vi "Sync2Tekron.vi"(0 "instrument handle in":refnum<k15>, 1 "error in (no error)":errorcluster) -> (7 "instrument handle out":refnum<k15>, 8 "error out":errorcluster, 9 "Synchronized":bool, 10 "Grandmaster Clock ID":string)   [LabVIEW 2021]
panel:
  in  "BMCA Mode":i32(ring) items=["SlaveOnly", "MasterSlave"]
  in  "1588:Clock Accuracy":i32(ring) items=["Unknown", "Within25nsec", "Within100nsec", "Within250nsec", "Within1usec", "Within2500nsec", "Within10usec", "Within25usec", "Within100usec", "Within250usec", "Within1msec", "Within2500usec", "Within10msec", "Within25msec", "Within100msec", "Within250msec", "Within1sec", "Within10sec", "GreaterThan10sec"]
  in  "Clock State":i32(ring) items=["Initializing", "Faulty", "Disabled", "Listening", "PreMaster", "Master", "Passive", "Uncalibrated", "Slave", "Stopped"]
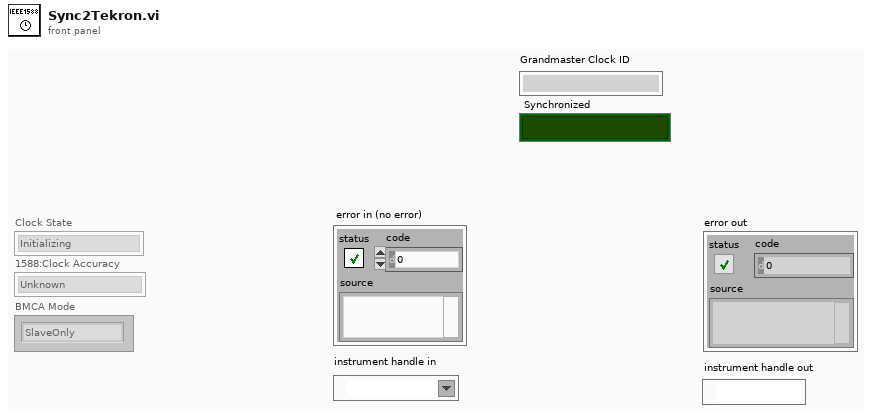
[diagram p1: front panel]
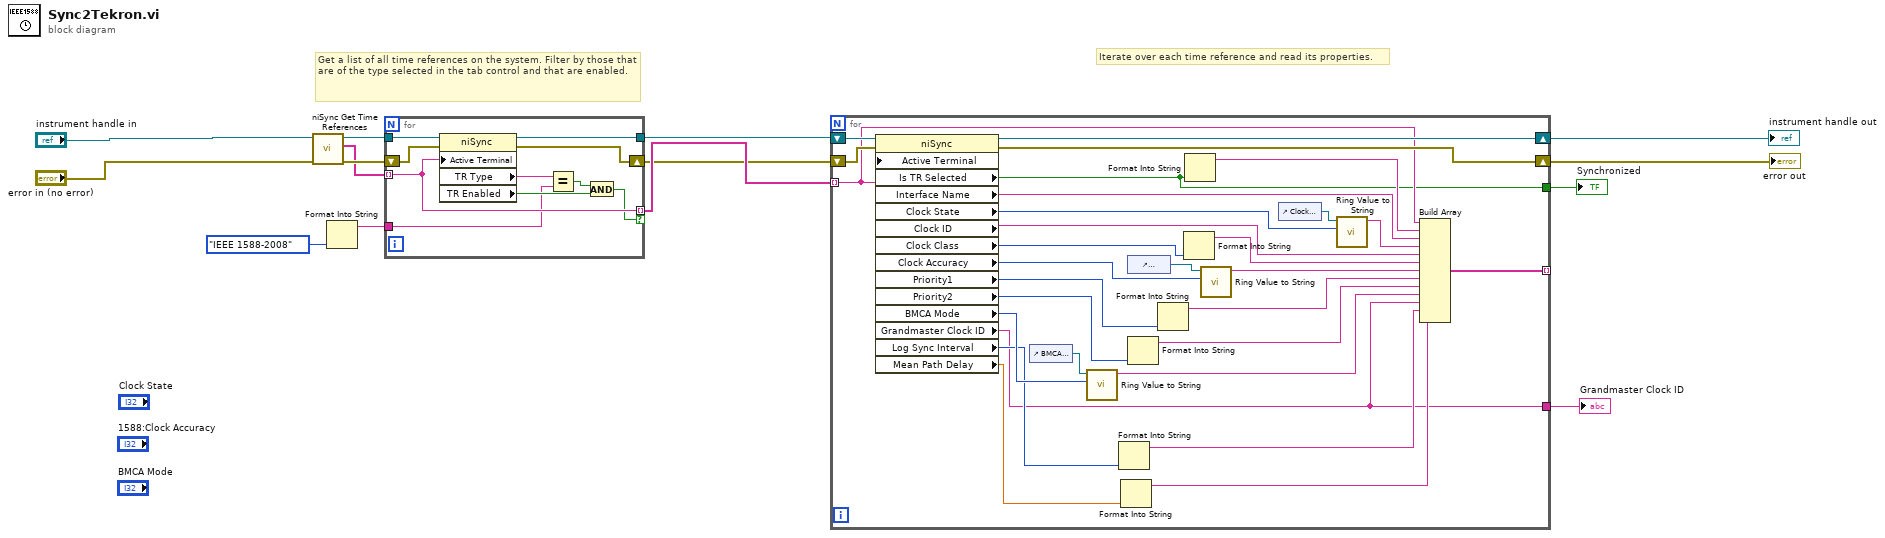
[diagram p0: block diagram]
diagram:
  # "Iterate over each time reference and read its properties."
  # "Get a list of all time references on the system. Filter by those that are of the type selected in the tab control and that are enabled."
  n1 = call <instrlib>:"niSync Get Time References.vi"("error in (no error)"="error in (no error)", "instrument handle"="instrument handle in") -> ("error out"=w13:errorcluster, "time references"=w12:string[], "instrument handle out"=w14:refnum<k15>)  [unwired: 7 in]
  n2 = Format Into String(enum32{"IEEE 1588-2008", "IEEE 802.1AS-2011"}."IEEE 1588-2008" ("input 1")) -> (resulting string=w9:string)  [unwired: 3 in, 1 out]
  n3 = for {
    tunnel: w14 -> [w24]
    tunnel: w12 -> [w21] mode=indexing
    tunnel: w9 -> [w15]
    tunnel: [w21] -> w11 mode=indexing if=w17
    tunnel: [w20] -> w5
    shift-right: [w16] -> w10
    shift-left: w13 -> [w23]
    n4 = property class="niSync"(reference=w24, error in=w23, "Active Terminal"=w21) -> (reference out=w20:refnum<k15>, error out=w16:errorcluster, "TR Type"=w22:string, "TR Enabled"=w18:bool)
    n5 = Equal?(x=w22, y=w15) -> (x = y?=w19:bool)
    n6 = And(x=w19, y=w18) -> (x .and. y?=w17:bool)
  }
  n7 = for {
    tunnel: w11 -> [w32] mode=indexing
    shift-right: [w35] -> w6
    shift-left: w10 -> [w52]
    tunnel: [w51] -> _ mode=indexing
    shift-right: [w53] -> w1
    shift-left: w5 -> [w54]
    tunnel: [w26] -> w7
    tunnel: [w25] -> w8
    n8 = property class="niSync"(reference=w54, error in=w52, "Active Terminal"=w32) -> (reference out=w53:refnum<k15>, error out=w35:errorcluster, "Is TR Selected"=w25:bool, "Interface Name"=w34:string, "Clock State"=w47:i32, "Clock ID"=w45:string, "Clock Class"=w50:i32, "Clock Accuracy"=w49:i32, "Priority1"=w48:i32, "Priority2"=w39:i32, "BMCA Mode"=w38:i32, "Grandmaster Clock ID"=w26:string, "Log Sync Interval"=w30:i32, "Mean Path Delay"=w28:dbl)
    n9 = control-ref of="BMCA Mode"() -> (w31:refnum<vi>)
    n10 = call "Ring Value to String.vi"("Value"=w38, "Ring in"=w31) -> ("String"=w37:string)  [unwired: 9 in]
    n11 = Format Into String(w30) -> (resulting string=w29:string)  [unwired: 3 in, 1 out]
    n12 = Format Into String(w28) -> (resulting string=w27:string)  [unwired: 3 in, 1 out]
    n13 = control-ref of="1588:Clock Accuracy"() -> (w40:refnum<vi>)
    n14 = Format Into String(w39) -> (resulting string=w41:string)  [unwired: 3 in, 1 out]
    n15 = Format Into String(w48) -> (resulting string=w42:string)  [unwired: 3 in, 1 out]
    n16 = Format Into String(w50) -> (resulting string=w44:string)  [unwired: 3 in, 1 out]
    n17 = Format Into String(w25) -> (resulting string=w33:string)  [unwired: 3 in, 1 out]
    n18 = call "Ring Value to String.vi"("Value"=w49, "Ring in"=w40) -> ("String"=w43:string)  [unwired: 9 in]
    n19 = control-ref of="Clock State"() -> (w36:refnum<vi>)
    n20 = call "Ring Value to String.vi"("Value"=w47, "Ring in"=w36) -> ("String"=w46:string)  [unwired: 9 in]
    n21 = Build Array(w32, w33, w34, w46, w45, w44, w43, w42, w41, w37, w26, w29, w27) -> (w51:string[])
  }
  "Grandmaster Clock ID" <- w7
  "Synchronized" <- w8
  "instrument handle out" <- w1
  "error out" <- w6
